vi "Chan_by_UT.vi"(2 "UnitType 2":T1(ring)) -> (7 "Graph Strings [] 2":string[](array[string]), 9 "Ch Strings []":string[](array[string]))   [LabVIEW 2017]
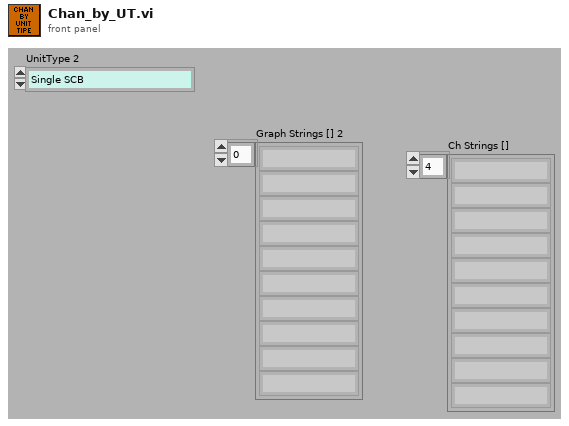
[diagram p1: front panel]
types:
  T1 = enum16{"Single SCB", "Power Rider", "Power Rider&Next10", "HATAL", "DAPH", "Indefinite", "Power Rider 12"}
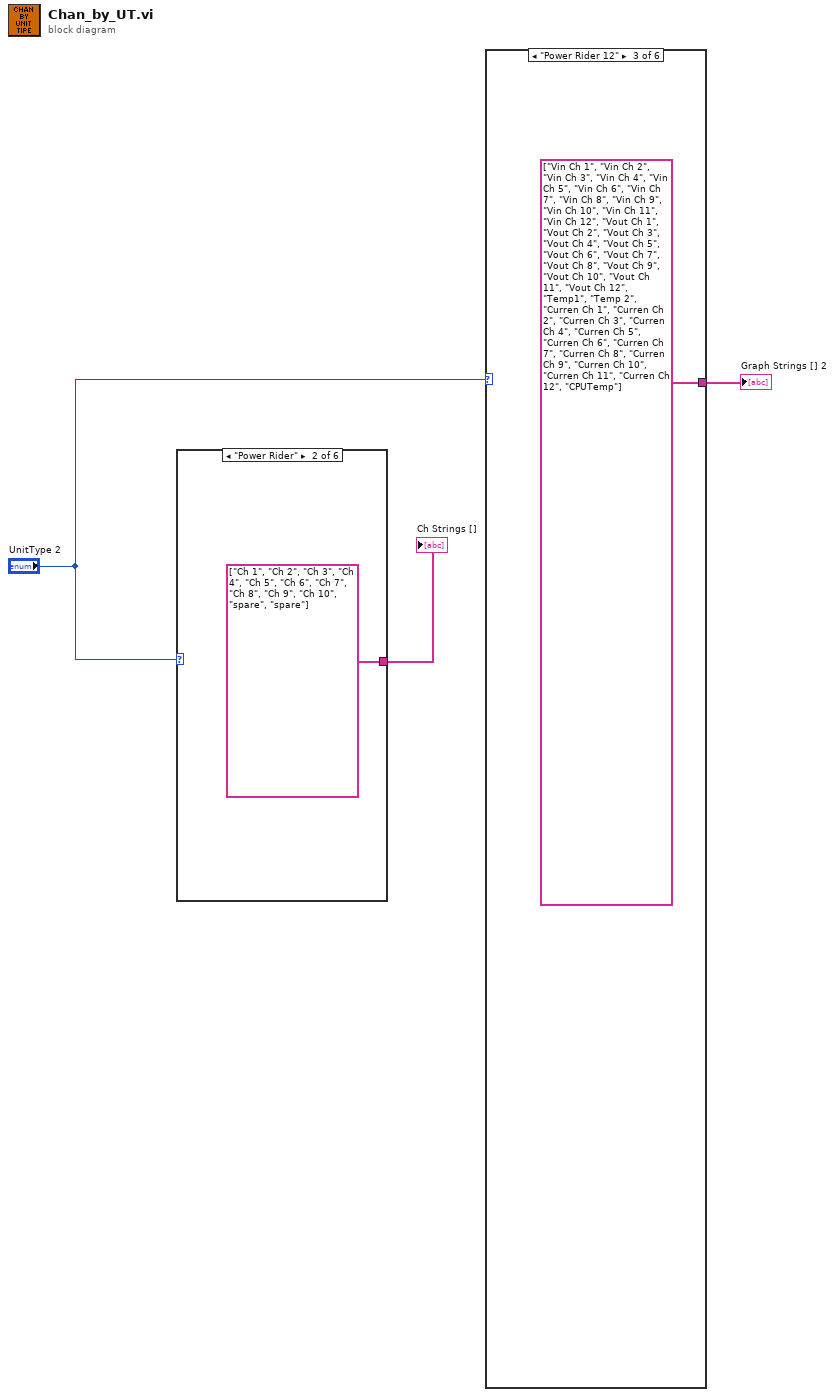
[diagram p0: block diagram]
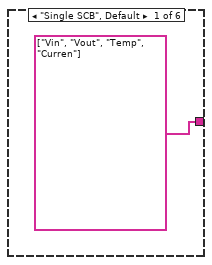
[diagram p2: hidden frame]
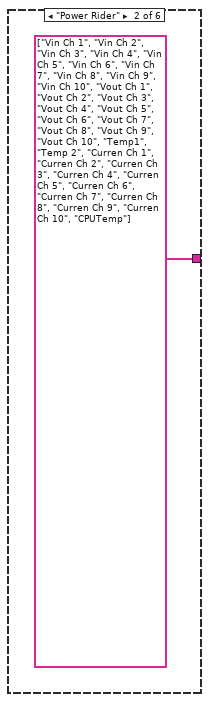
[diagram p3: hidden frame]
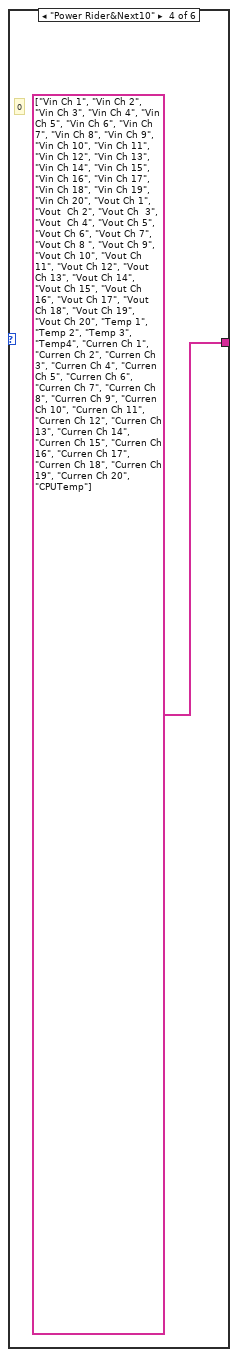
[diagram p4: hidden frame]
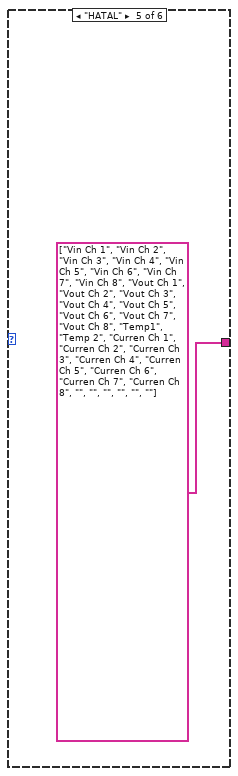
[diagram p5: hidden frame]
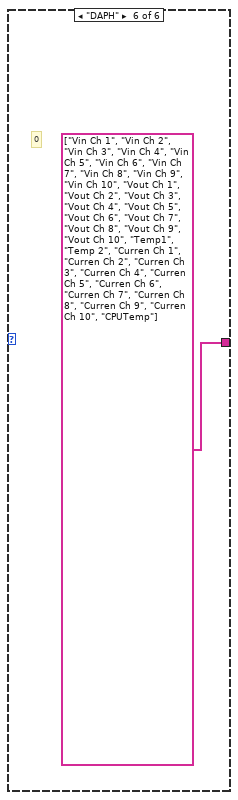
[diagram p6: hidden frame]
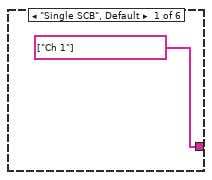
[diagram p7: hidden frame]
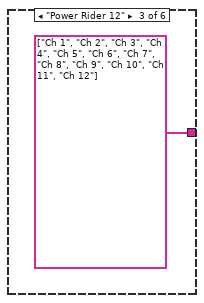
[diagram p8: hidden frame]
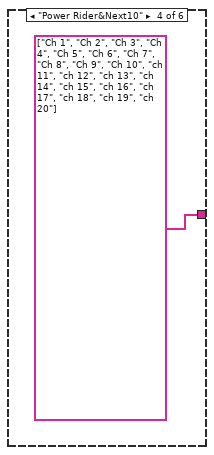
[diagram p9: hidden frame]
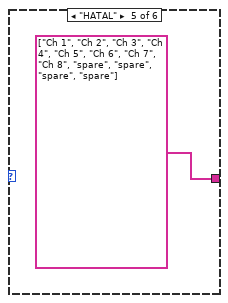
[diagram p10: hidden frame]
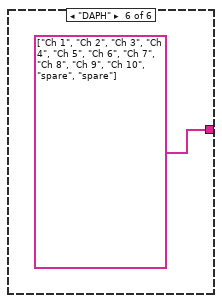
[diagram p11: hidden frame]
diagram:
  n1 = case shown="\"Power Rider\"" "UnitType 2" {
    tunnel: [string[] ["Ch 1"] ("Strings []") string[] ["Ch 1", "Ch 2", "Ch 3", "Ch 4", "Ch 5", "Ch 6", "Ch 7", "Ch 8", "Ch 9", "Ch 10", "spare", "spare"] ("Strings []") string[] ["Ch 1", "Ch 2", "Ch 3", "Ch 4", "Ch 5", "Ch 6", "Ch 7", "Ch 8", "Ch 9", "Ch 10", "Ch 11", "Ch 12"] ("Strings []") string[] ["Ch 1", "Ch 2", "Ch 3", "Ch 4", "Ch 5", "Ch 6", "Ch 7", "Ch 8", "Ch 9", "Ch 10", "ch 11", "ch 12", "ch 13", "ch 14", "ch 15", "ch 16", "ch 17", "ch 18", "ch 19", "ch 20"] ("Strings []") string[] ["Ch 1", "Ch 2", "Ch 3", "Ch 4", "Ch 5", "Ch 6", "Ch 7", "Ch 8", "spare", "spare", "spare", "spare"] ("Strings []") string[] ["Ch 1", "Ch 2", "Ch 3", "Ch 4", "Ch 5", "Ch 6", "Ch 7", "Ch 8", "Ch 9", "Ch 10", "spare", "spare"] ("Strings []")] -> w3
    frame "Single SCB", Default {
    }
    frame "Power Rider" {
    }
    frame "Power Rider 12" {
    }
    frame "Power Rider&Next10" {
    }
    frame "HATAL" {
    }
    frame "DAPH" {
    }
  }
  "Ch Strings []" <- w3
  n2 = case shown="\"Power Rider 12\"" "UnitType 2" {
    tunnel: [string[] ["Vin", "Vout", "Temp", "Curren"] ("Strings []") string[] ["Vin Ch 1", "Vin Ch 2", "Vin Ch 3", "Vin Ch 4", "Vin Ch 5", "Vin Ch 6", "Vin Ch 7", "Vin Ch 8", "Vin Ch 9", "Vin Ch 10", "Vout Ch 1", "Vout Ch 2", "Vout Ch 3", "Vout Ch 4", "Vout Ch 5", "Vout Ch 6", "Vout Ch 7", "Vout Ch 8", "Vout Ch 9", "Vout Ch 10", "Temp1", "Temp 2", "Curren Ch 1", "Curren Ch 2", "Curren Ch 3", "Curren Ch 4", "Curren Ch 5", "Curren Ch 6", "Curren Ch 7", "Curren Ch 8", "Curren Ch 9", "Curren Ch 10", "CPUTemp"] ("Strings []") string[] ["Vin Ch 1", "Vin Ch 2", "Vin Ch 3", "Vin Ch 4", "Vin Ch 5", "Vin Ch 6", "Vin Ch 7", "Vin Ch 8", "Vin Ch 9", "Vin Ch 10", "Vin Ch 11", "Vin Ch 12", "Vout Ch 1", "Vout Ch 2", "Vout Ch 3", "Vout Ch 4", "Vout Ch 5", "Vout Ch 6", "Vout Ch 7", "Vout Ch 8", "Vout Ch 9", "Vout Ch 10", "Vout Ch 11", "Vout Ch 12", "Temp1", "Temp 2", "Curren Ch 1", "Curren Ch 2", "Curren Ch 3", "Curren Ch 4", "Curren Ch 5", "Curren Ch 6", "Curren Ch 7", "Curren Ch 8", "Curren Ch 9", "Curren Ch 10", "Curren Ch 11", "Curren Ch 12", "CPUTemp"] ("Strings []") string[] ["Vin Ch 1", "Vin Ch 2", "Vin Ch 3", "Vin Ch 4", "Vin Ch 5", "Vin Ch 6", "Vin Ch 7", "Vin Ch 8", "Vin Ch 9", "Vin Ch 10", "Vin Ch 11", "Vin Ch 12", "Vin Ch 13", "Vin Ch 14", "Vin Ch 15", "Vin Ch 16", "Vin Ch 17", "Vin Ch 18", "Vin Ch 19", "Vin Ch 20", "Vout Ch 1", "Vout  Ch 2", "Vout Ch  3", "Vout  Ch 4", "Vout Ch 5", "Vout Ch 6", "Vout Ch 7", "Vout Ch 8 ", "Vout Ch 9", "Vout Ch 10", "Vout Ch 11", "Vout Ch 12", "Vout Ch 13", "Vout Ch 14", "Vout Ch 15", "Vout Ch 16", "Vout Ch 17", "Vout Ch 18", "Vout Ch 19", "Vout Ch 20", "Temp 1", "Temp 2", "Temp 3", "Temp4", "Curren Ch 1", "Curren Ch 2", "Curren Ch 3", "Curren Ch 4", "Curren Ch 5", "Curren Ch 6", "Curren Ch 7", "Curren Ch 8", "Curren Ch 9", "Curren Ch 10", "Curren Ch 11", "Curren Ch 12", "Curren Ch 13", "Curren Ch 14", "Curren Ch 15", "Curren Ch 16", "Curren Ch 17", "Curren Ch 18", "Curren Ch 19", "Curren Ch 20", "CPUTemp"] ("Strings []") string[] ["Vin Ch 1", "Vin Ch 2", "Vin Ch 3", "Vin Ch 4", "Vin Ch 5", "Vin Ch 6", "Vin Ch 7", "Vin Ch 8", "Vout Ch 1", "Vout Ch 2", "Vout Ch 3", "Vout Ch 4", "Vout Ch 5", "Vout Ch 6", "Vout Ch 7", "Vout Ch 8", "Temp1", "Temp 2", "Curren Ch 1", "Curren Ch 2", "Curren Ch 3", "Curren Ch 4", "Curren Ch 5", "Curren Ch 6", "Curren Ch 7", "Curren Ch 8", "", "", "", "", "", ""] ("Strings []") string[] ["Vin Ch 1", "Vin Ch 2", "Vin Ch 3", "Vin Ch 4", "Vin Ch 5", "Vin Ch 6", "Vin Ch 7", "Vin Ch 8", "Vin Ch 9", "Vin Ch 10", "Vout Ch 1", "Vout Ch 2", "Vout Ch 3", "Vout Ch 4", "Vout Ch 5", "Vout Ch 6", "Vout Ch 7", "Vout Ch 8", "Vout Ch 9", "Vout Ch 10", "Temp1", "Temp 2", "Curren Ch 1", "Curren Ch 2", "Curren Ch 3", "Curren Ch 4", "Curren Ch 5", "Curren Ch 6", "Curren Ch 7", "Curren Ch 8", "Curren Ch 9", "Curren Ch 10", "CPUTemp"] ("Strings []")] -> w2
    frame "Single SCB", Default {
    }
    frame "Power Rider" {
    }
    frame "Power Rider 12" {
    }
    frame "Power Rider&Next10" {
      # "63"
      # "44"
      # "43"
      # "40"
      # "39"
      # "20"
      # "19"
      # "0"
    }
    frame "HATAL" {
      # "25"
      # "18"
      # "16"
      # "17"
      # "15"
      # "8"
      # "7"
    }
    frame "DAPH" {
      # "31"
      # "22"
      # "20"
      # "21"
      # "19"
      # "10"
      # "9"
      # "0"
    }
  }
  "Graph Strings [] 2" <- w2
